vi "HO3_1.vi"() -> ()   [LabVIEW 2020]
panel:
  out "Time Stamp":timestamp
  out "age":string
  out "Birthday":string
  out "Current Time":string
  in  "Contact":T1={"First Name"="", "Last Name"="", "Birthday"=timestamp(61200.46228170395 s since 1904-01-01), "Age"=0.0, "Favorite"=FALSE} {"Birthday" format="%<%x>T"}
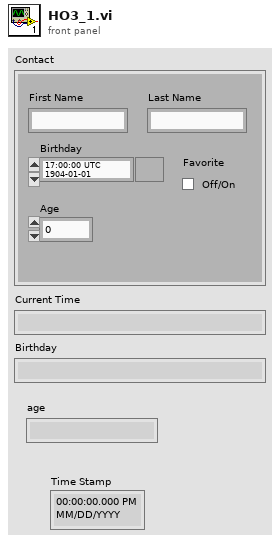
[diagram p1: front panel]
types:
  T1 = cluster{"First Name":string, "Last Name":string, "Birthday":timestamp, "Age":dbl, "Favorite":bool}
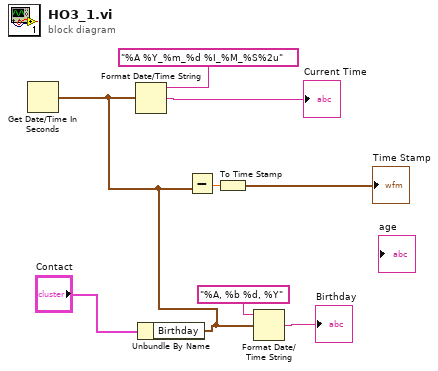
[diagram p0: block diagram]
diagram:
  n1 = Get Date/Time In Seconds() -> (seconds since 1Jan1904=w1:timestamp)
  n2 = Format Date/Time String(time format string (%c)="%A %Y_%m_%d %I_%M_%S%2u", seconds (now)=w1) -> (date/time string=→"Current Time":string)  [unwired: 1 in]
  n3 = Unbundle By Name("Contact", "Birthday"=w1) -> ()
  n4 = Subtract(y=w1) -> (x-y=w2:dbl)  [unwired: 1 in]
  n5 = To Time Stamp(1:w2) -> (0:→"Time Stamp":timestamp)
  n6 = Format Date/Time String(time format string (%c)="%A, %b %d, %Y", seconds (now)=w1) -> (date/time string=→"Birthday":string)  [unwired: 1 in]
